vi "data_Close Notifiers.vi"(8 "error in":errorcluster, 11 "Data Notifiers":T1) -> (0 "error out":errorcluster)   [LabVIEW 2017]
uses:
  data_Notifiers.ctl
  measurement_data/MeasurementDatalvclass.lvclass
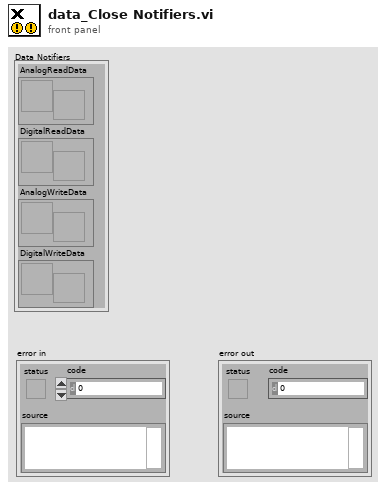
[diagram p1: front panel]
types:
  T1 = typedef "data_Notifiers.ctl" = cluster{"AnalogReadData":refnum<notifier>, "DigitalReadData":refnum<notifier>, "AnalogWriteData":refnum<notifier>, "DigitalWriteData":refnum<notifier>}
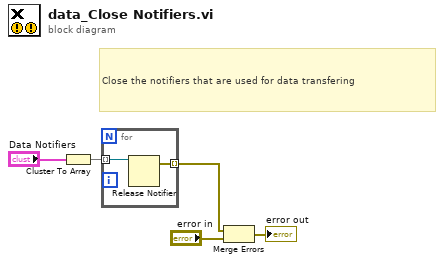
[diagram p0: block diagram]
diagram:
  # "Close the notifiers that are used for data transfering"
  n1 = Cluster To Array(cluster="Data Notifiers") -> (array=w4:refnum<notifier>[])
  n2 = for {
    tunnel: w4 -> [w7] mode=indexing
    tunnel: [w6] -> w3 mode=indexing
    n3 = Release Notifier(notifier=w7) -> (error out=w6:errorcluster)  [unwired: 2 in, 2 out]
  }
  n4 = Merge Errors(w3, "error in") -> (→"error out":errorcluster)
